vi "ToText.vi"(8 "error in":errorcluster, 11 "Generic":refnum<class "Generic.lvclass">) -> (0 "error out":errorcluster, 3 "Text out":refnum<class "Text.lvclass">)   [LabVIEW 2014, in "Text.lvclass"]
uses:
  Text.lvclass
  Generic/Generic.lvclass
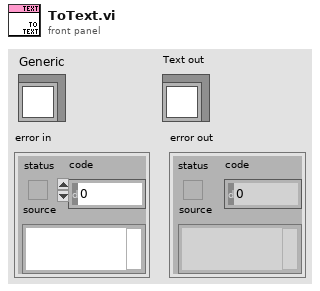
[diagram p1: front panel]
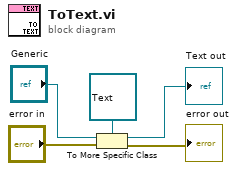
[diagram p0: block diagram]
diagram:
  n1 = To More Specific Class(target class=refnum<class "Text.lvclass"> refnum ("Text out"), reference="Generic", error in="error in") -> (specific class reference=→"Text out":refnum<class "Text.lvclass">, error out=→"error out":errorcluster)
